vi "Return Panel Info.vi"(6 "Data":variant, 7 "VI Running Refnum":refnum<vi>, 8 "error in (no error)":errorcluster, 9 "Panel VI Path":path, 10 "Console_Q":refnum<class "Message Enqueuer.lvclass">, 11 "Console2API Q in":refnum<class "Console Reply.lvclass">) -> (0 "error out":errorcluster, 3 "Console2API Q out":refnum<class "Console Reply.lvclass">)   [LabVIEW 2015]
uses:
  Console Reply.lvclass
  <vilib>/ActorFramework/Message Enqueuer/Message Enqueuer.lvclass
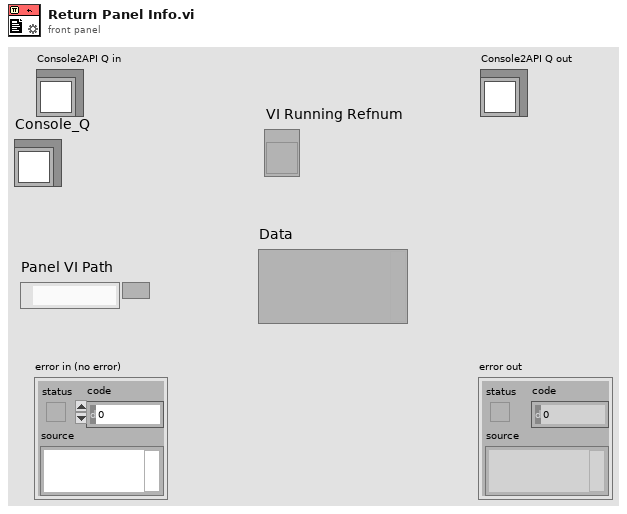
[diagram p1: front panel]
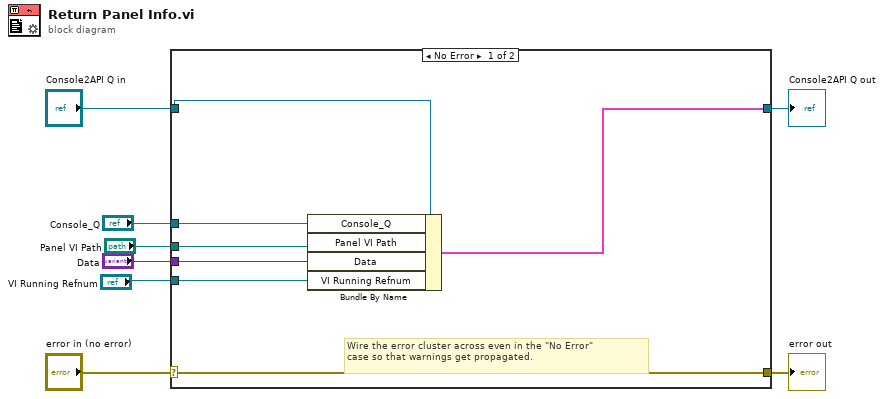
[diagram p0: block diagram]
diagram:
  n1 = case shown="No Error" "error in (no error)" {
    selector: "error in (no error)" -> [w15 w17]
    tunnel: [w15 w17] -> w7
    tunnel: [w13 w16] -> w5
    tunnel: "Console2API Q in" -> [w14 w16]
    tunnel: "Console_Q" -> [w12 _]
    tunnel: "Panel VI Path" -> [w11 _]
    tunnel: "Data" -> [w10 _]
    tunnel: "VI Running Refnum" -> [w9 _]
    frame No Error {
      # "Wire the error cluster across even in the \"No Error\"\ncase so that warnings get propagated."
      n2 = Bundle By Name(cluster=w14, "Console_Q"=w12, "Panel VI Path"=w11, "Data"=w10, "VI Running Refnum"=w9) -> (w13:cluster{})
    }
    frame Error {
    }
  }
  "error out" <- w7
  "Console2API Q out" <- w5
